vi "Save Stabilisation Data.vi"(0 "Experiment Indicator":string, 1 "Cell details cluster":T1={"Cell Position"=16, "Cell Label"="", "Pixel to measure"=0, "Area (cm^2)"=0.126, "Variable"="", "Variable value"="", "Scan settings in queue"=0, "Light or dark"="", "Measurement Type"=""} {"Pixel to measure" items=["All", "1", "2", "3", "4", "5", "6", "7", "8"]}, 3 "Intensity (no. of suns)":string, 4 "Data Array":dbl[][](array[numeric]), 6 "Username":string, 10 "Date array":string[](array[string])) -> (17 "File path for Jt data":path, 18 "File path for Jt image":path)   [LabVIEW 2011]
uses:
  <vilib>/Utility/file.llb/Write To Spreadsheet File (string).vi
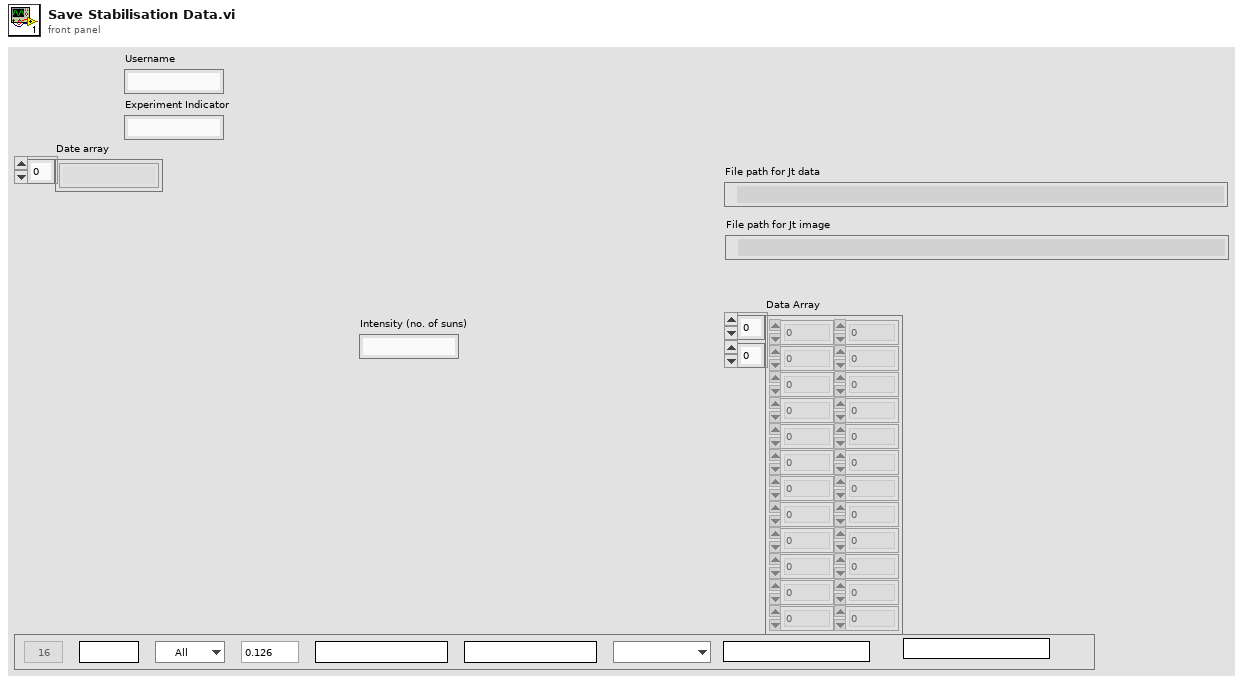
[diagram p1: front panel]
types:
  T1 = cluster{"Cell Position":i32, "Cell Label":string, "Pixel to measure":u16, "Area (cm^2)":dbl, "Variable":string, "Variable value":string, "Scan settings in queue":u16, "Light or dark":string, "Measurement Type":string}
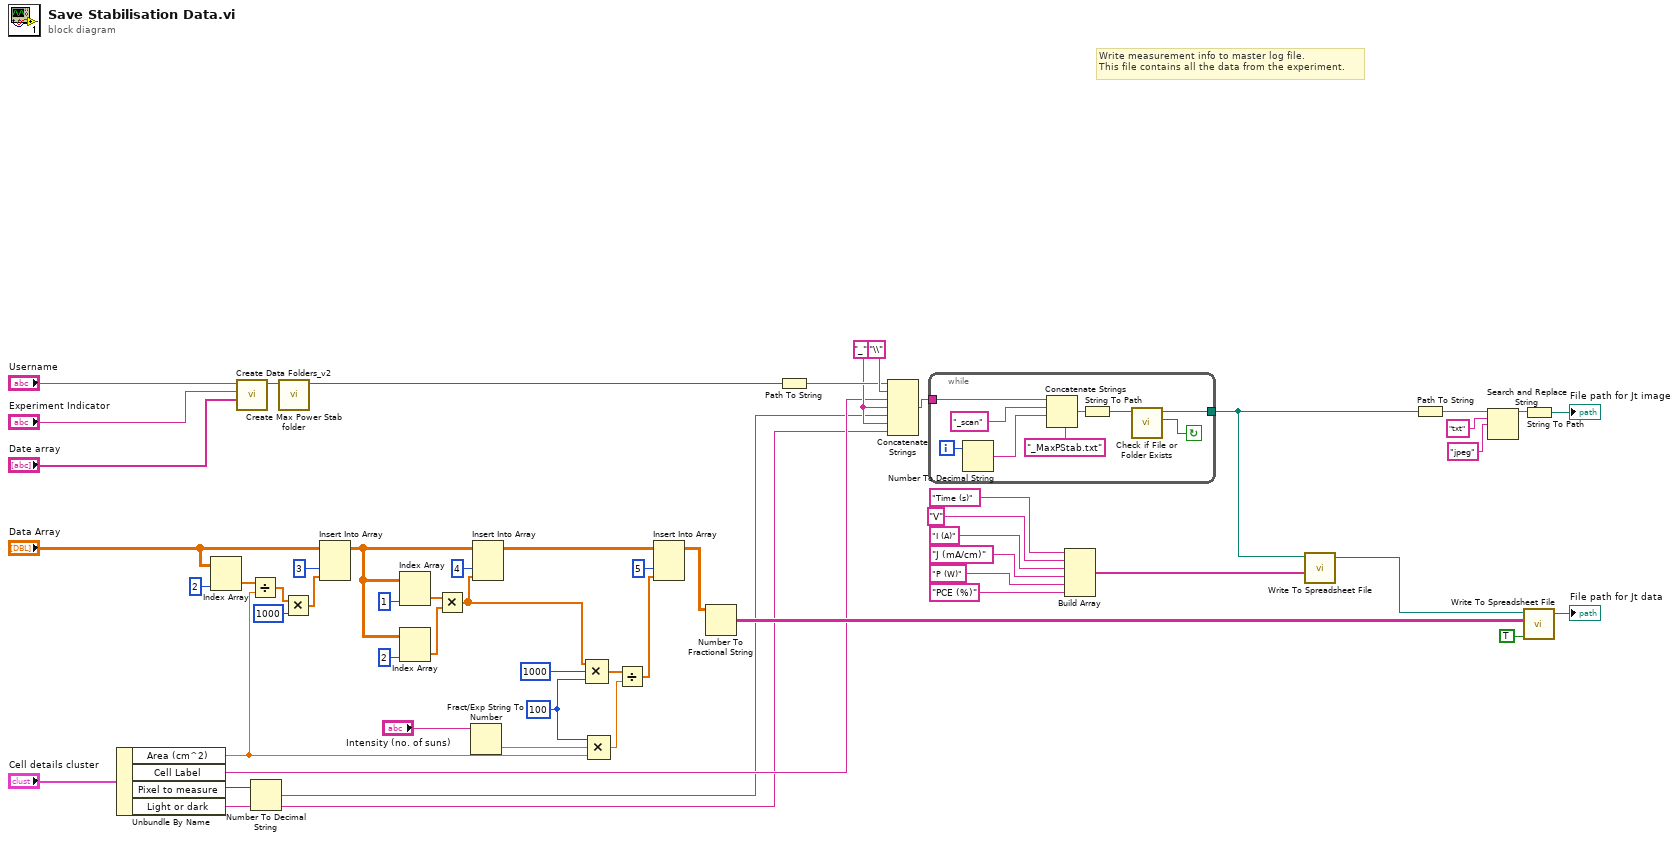
[diagram p0: block diagram]
diagram:
  w13 = 100
  w45 = "_"
  # "Write measurement info to master log file.\nThis file contains all the data from the experiment."
  n1 = Unbundle By Name("Cell details cluster") -> ("Area (cm^2)"=w12:dbl, "Cell Label"=w40:string, "Pixel to measure"=w38:u16, "Light or dark"=w39:string)
  n2 = Index Array(array="Data Array", index (col)=2) -> (element=w43:dbl[])  [unwired: 1 in]
  n3 = call "Create Data Folders_v2.vi"("Date array"="Date array", "Experiment Indicator"="Experiment Indicator", "username"="Username") -> ("Data Output Folder"=w2:path)  [unwired: 8 in]
  n4 = Divide(x=w43, y=w12) -> (x/y=w35:dbl[])
  n5 = Number To Decimal String(number=w38) -> (decimal integer string=w37:string)  [unwired: 1 in]
  n6 = call "Create Max Power Stab folder.vi"("Data Folder In"=w2) -> ("Data Output Folder"=w3:path)  [unwired: 10 in]
  n7 = Multiply(x=w35, y=1000) -> (x*y=w36:dbl[])
  n8 = Insert Into Array(array="Data Array", index (col)=3, new element=w36) -> (w19:dbl[][])  [unwired: 1 in]
  n9 = Index Array(array=w19, index (col)=1 ("disabled index (col)")) -> (element=w24:dbl[])  [unwired: 1 in]
  n10 = Index Array(array=w19, index (col)=2 ("disabled index (col)")) -> (element=w23:dbl[])  [unwired: 1 in]
  n11 = Multiply(x=w24, y=w23) -> (x*y=w4:dbl[])
  n12 = Fract/Exp String To Number(string="Intensity (no. of suns)") -> (number=w11:dbl)  [unwired: 3 in, 1 out]
  n13 = Insert Into Array(array=w19, index (col)=4 ("disabled index (col)"), new element=w4) -> (w18:dbl[][])  [unwired: 1 in]
  n14 = Compound Arithmetic op=MULTIPLY(w4, 1000, w13) -> (w14:dbl[])
  n15 = Compound Arithmetic op=MULTIPLY(w13, w11, w12) -> (w10:dbl)
  n16 = Divide(x=w14, y=w10) -> (x/y=w9:dbl[])
  n17 = Insert Into Array(array=w18, index (col)=5 ("disabled index (col)"), new element=w9) -> (w8:dbl[][])  [unwired: 1 in]
  n18 = Number To Fractional String(number=w8) -> (F-format string=w44:string[][])  [unwired: 3 in]
  n19 = Path To String(path=w3) -> (string=w55:string)
  n20 = Concatenate Strings(w55, "\\", w40, w45, w37, w45, w39) -> (w47:string)
  n21 = while {
    tunnel: w47 -> [w65]
    tunnel: [w57] -> w33
    i -> [w63]
    stop <- w58 continue-if-true
    n22 = Number To Decimal String(number=w63) -> (decimal integer string=w62:string)  [unwired: 1 in]
    n23 = Concatenate Strings(w65, "_scan", w62, "_MaxPStab.txt") -> (w59:string)
    n24 = String To Path(string=w59) -> (path=w60:path)
    n25 = call <vilib>:"Check if File or Folder Exists.vi"("path"=w60) -> ("file or folder exists?"=w58:bool, "dup path"=w57:path)  [unwired: 8 in, 1 out]
  }
  n26 = Build Array("Time (s)", "V", "I (A)", "J (mA/cm)", "P (W)", "PCE (%)") -> (w28:string[])
  n27 = call-poly <vilib>:"Write To Spreadsheet File.vi"("1D data"=w28, "file path (dialog if empty)"=w33) -> ("new file path (Not A Path if cancelled)"=w32:path)  [unwired: 6 in]
  n28 = Path To String(path=w33) -> (string=w46:string)
  n29 = Search and Replace String(input string=w46, search string="txt", replace string="jpeg") -> (result string=w54:string)  [unwired: 5 in, 3 out]
  n30 = String To Path(string=w54) -> (path=→"File path for Jt image":path)
  n31 = call-poly <vilib>:"Write To Spreadsheet File.vi"("append to file? (new file:F)"=TRUE, "2D data"=w44, "file path (dialog if empty)"=w32) -> ("new file path (Not A Path if cancelled)"=→"File path for Jt data":path)  [unwired: 5 in]
